vi "Untitled 4.vi"() -> ()   [LabVIEW 2019, in "Git.lvclass"]
uses:
  Git.lvclass
  Git.lvclass/Git.ctl
  <vilib>/JKI/VIPM API/VIPM API_vipm_api.lvlib
  VIPM/VIPM.lvlib
panel:
  in  "error in (no error)":errorcluster
  in  "Git.lvclass":refnum<class "Git.lvclass">
  out "input cluster":refnum<class "Git.lvclass">
  in  "Build Path":path
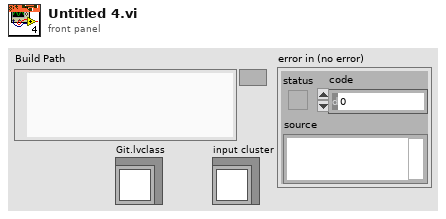
[diagram p1: front panel]
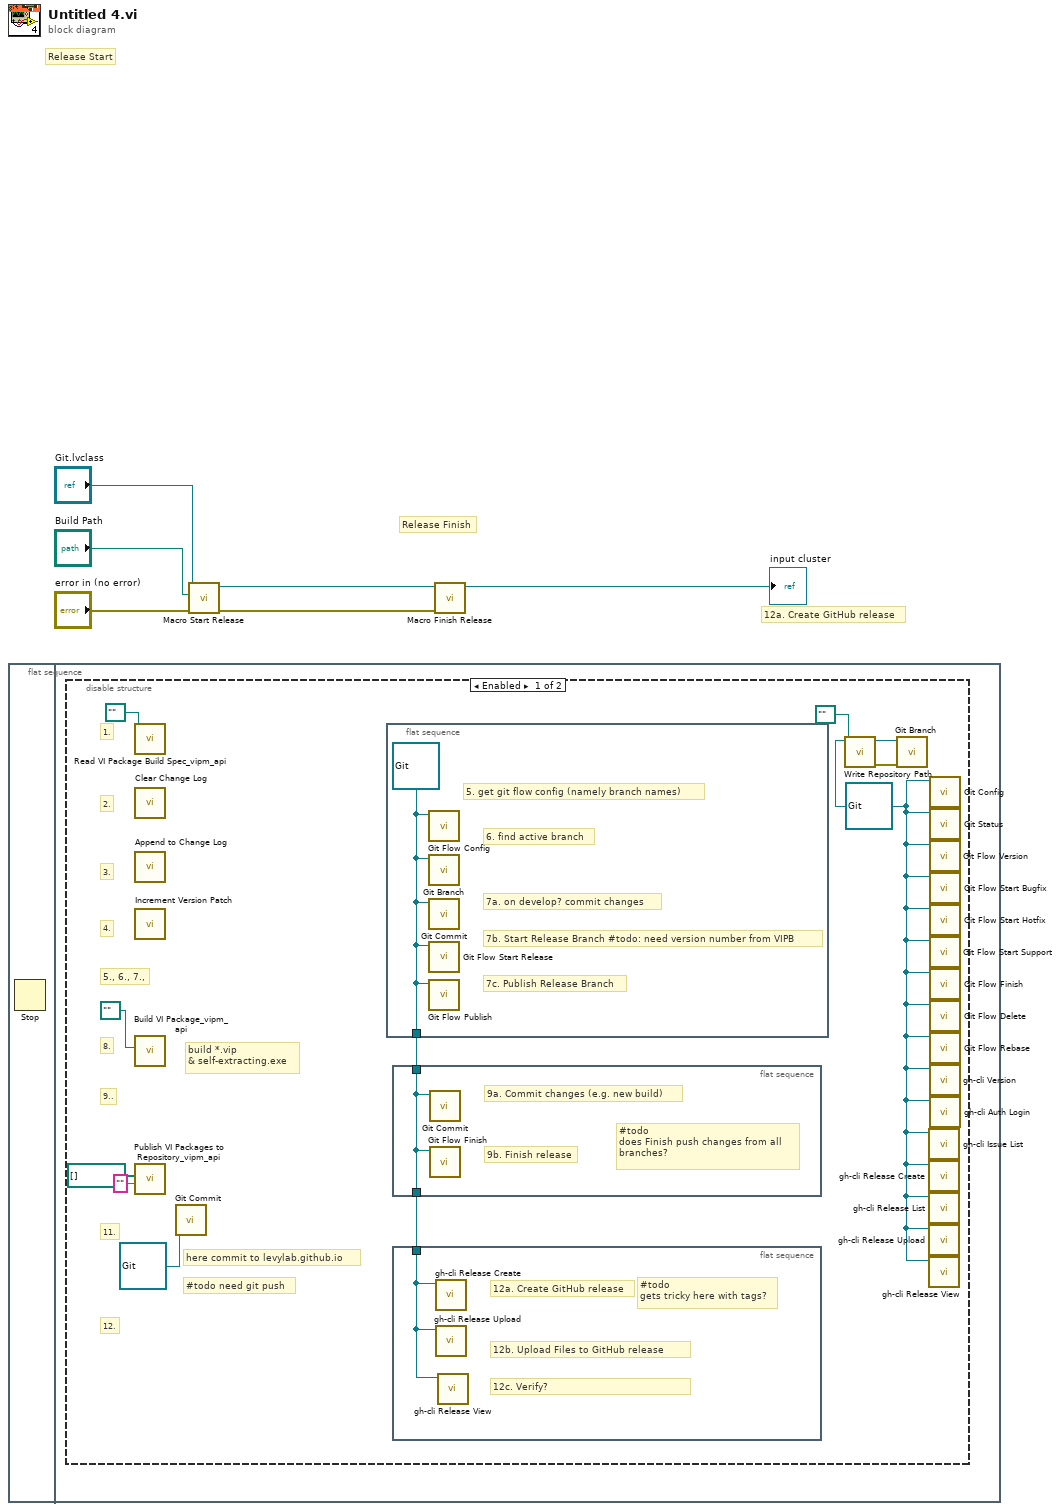
[diagram p0: block diagram]
diagram:
  # "12a. Create GitHub release"
  # "Release Finish"
  # "Release Start"
  n1 = flat-sequence {
    frame #0 {
      n2 = Stop() -> ()  [unwired: 1 in]
    }
    frame #1 {
      n3 = disable-structure shown="Enabled" {
        frame Enabled {
          w8 = refnum<class "Git.lvclass"> refnum ("Git in")
          # "build *.vip\n& self-extracting.exe"
          # "11."
          # "10."
          # "8."
          # "3."
          # "2."
          # "4."
          # "1."
          # "#todo need git push"
          # "here commit to levylab.github.io"
          # "12."
          # "9.."
          # "5., 6., 7.,"
          n4 = call <vilib>:"Read VI Package Build Spec_vipm_api.vi"("Path to VIPB File"=path "") -> ()  [unwired: 9 in, 2 out]
          n5 = call "Clear Change Log.vi"() -> ()  [unwired: 10 in, 2 out]
          n6 = call "Append to Change Log.vi"() -> ()  [unwired: 10 in, 2 out]
          n7 = call "Increment Version Patch.vi"() -> ()  [unwired: 10 in, 2 out]
          n8 = call <vilib>:"Build VI Package_vipm_api.vi"("Path to VIPB File"=path "") -> ()  [unwired: 9 in, 2 out]
          n9 = call <vilib>:"Publish VI Packages to Repository_vipm_api.vi"("Repository Name"="", "Packages to publish to Repository Library (vip,ogp)"=path[] []) -> ()  [unwired: 8 in, 2 out]
          n10 = call "Git Commit.vi"("Git in"=refnum<class "Git.lvclass"> refnum) -> ()  [unwired: 8 in, 3 out]
          n11 = flat-sequence {
            tunnel: [w20] -> w15
            frame #0 {
              w20 = refnum<class "Git.lvclass"> refnum ("Git in")
              # "7c. Publish Release Branch"
              # "7b. Start Release Branch #todo: need version number from VIPB"
              # "7a. on develop? commit changes"
              # "6. find active branch"
              # "5. get git flow config (namely branch names)"
              n12 = call "Git Flow Config.vi"("Git in"=w20) -> ()  [unwired: 8 in, 3 out]
              n13 = call "Git Branch.vi"("Git in"=w20) -> ()  [unwired: 7 in, 4 out]
              n14 = call "Git Commit.vi"("Git in"=w20) -> ()  [unwired: 8 in, 3 out]
              n15 = call "Git Flow Start Release.vi"("Git in"=w20) -> ()  [unwired: 8 in, 3 out]
              n16 = call "Git Flow Publish.vi"("Git in"=w20) -> ()  [unwired: 8 in, 3 out]
            }
          }
          n17 = flat-sequence {
            tunnel: w15 -> [w19]
            tunnel: [w19] -> w14
            frame #0 {
              # "#todo\ndoes Finish push changes from all\nbranches?"
              # "9a. Commit changes (e.g. new build)"
              # "9b. Finish release"
              n18 = call "Git Commit.vi"("Git in"=w19) -> ()  [unwired: 8 in, 3 out]
              n19 = call "Git Flow Finish.vi"("Git in"=w19) -> ()  [unwired: 8 in, 3 out]
            }
          }
          n20 = flat-sequence {
            tunnel: w14 -> [w18]
            frame #0 {
              # "12c. Verify?"
              # "#todo\ngets tricky here with tags?"
              # "12a. Create GitHub release"
              # "12b. Upload Files to GitHub release"
              n21 = call "gh-cli Release Create.vi"("Git in"=w18) -> ()  [unwired: 8 in, 3 out]
              n22 = call "gh-cli Release Upload.vi"("Git in"=w18) -> ()  [unwired: 8 in, 3 out]
              n23 = call "gh-cli Release View.vi"("Git in"=w18) -> ()  [unwired: 8 in, 3 out]
            }
          }
          n24 = call "Write Repository Path.vi"("Repository Path"=path "", "Git in"=w8) -> ("error out"=w17:errorcluster, "Git out"=w16:refnum<class "Git.lvclass">)  [unwired: 8 in]
          n25 = call "Git Branch.vi"("error in (no error)"=w17, "Git in"=w16) -> ()  [unwired: 6 in, 4 out]
          n26 = call "gh-cli Issue List.vi"("Git in"=w8) -> ()  [unwired: 8 in, 3 out]
          n27 = call "gh-cli Release Create.vi"("Git in"=w8) -> ()  [unwired: 8 in, 3 out]
          n28 = call "gh-cli Release List.vi"("Git in"=w8) -> ()  [unwired: 8 in, 3 out]
          n29 = call "gh-cli Release Upload.vi"("Git in"=w8) -> ()  [unwired: 8 in, 3 out]
          n30 = call "gh-cli Release View.vi"("Git in"=w8) -> ()  [unwired: 8 in, 3 out]
          n31 = call "Git Config.vi"("Git in"=w8) -> ()  [unwired: 8 in, 3 out]
          n32 = call "Git Status.vi"("Git in"=w8) -> ()  [unwired: 8 in, 3 out]
          n33 = call "Git Flow Version.vi"("Git in"=w8) -> ()  [unwired: 8 in, 3 out]
          n34 = call "Git Flow Start Bugfix.vi"("Git in"=w8) -> ()  [unwired: 8 in, 3 out]
          n35 = call "Git Flow Start Hotfix.vi"("Git in"=w8) -> ()  [unwired: 8 in, 3 out]
          n36 = call "Git Flow Start Support.vi"("Git in"=w8) -> ()  [unwired: 8 in, 3 out]
          n37 = call "Git Flow Finish.vi"("Git in"=w8) -> ()  [unwired: 8 in, 3 out]
          n38 = call "Git Flow Delete.vi"("Git in"=w8) -> ()  [unwired: 8 in, 3 out]
          n39 = call "Git Flow Rebase.vi"("Git in"=w8) -> ()  [unwired: 8 in, 3 out]
          n40 = call "gh-cli Version.vi"("Git in"=w8) -> ()  [unwired: 8 in, 3 out]
          n41 = call "gh-cli Auth Login.vi"("Git in"=w8) -> ()  [unwired: 9 in, 2 out]
        }
        frame Disabled {
        }
      }
    }
  }
  n42 = call "Macro Start Release.vi"("error in (no error)"="error in (no error)", "VIPB Path"="Build Path", "Git in"="Git.lvclass") -> ("error out"=w5:errorcluster, "Git out"=w3:refnum<class "Git.lvclass">)  [unwired: 7 in]
  n43 = call "Macro Finish Release.vi"("error in (no error)"=w5, "Git in"=w3) -> ("Git out"=→"input cluster":refnum<class "Git.lvclass">)  [unwired: 7 in, 2 out]
